vi "Clear Filters.vi"(8 "error in (no error)":errorcluster, 11 "Local Error Manager in":refnum<class "Local Error Manager.lvclass">) -> (0 "error out":errorcluster, 2 "Filters to clear":set{i32}(c389), 3 "Local Error Manager out":refnum<class "Local Error Manager.lvclass">)   [LabVIEW 2026, in "TALOS.lvlib" / "Error Manager.lvlib" / "Local Error Manager.lvclass"]
uses:
  Local Error Manager.lvclass
  Ancestor/Ancestor/Ancestor.lvclass/Ancestor.ctl
  Support VIs/Generate Error.vi
  FGV/Error Memory/Get Error Description.vi
  Support VIs/Get PC name.vi
  Ancestor/Ancestor/Read ID.vi
  Support VIs/Get Class Name.vi
  <vilib>/Utility/error.llb/Clear Errors.vi
  FGV/Error Memory/Error Memory Core.vi
  <vilib>/AdvancedString/Delimited String to 1D String Array.vi
  <vilib>/AdvancedString/Delimited String to 1D String Array (string).vi
  Support VIs/Circus Root Path.vi
  FGV/Error Memory/Error Crt Lvl checker.vi
  FGV/Error Memory/Error Memory Core.vi/40c8088d-b597-4017-91af-faa98e00292e.vi
  FGV/Error Memory/Error Memory Core.vi/d4a3ab98-063c-4e44-b43d-fbdcfe6c2be2.vi
  Support VIs/Global Memory.vi
  <vilib>/Utility/LVClass/Get LV Class Name.vi
  Support VIs/Is in Packed Library.vi
  Support VIs/TALOS Root path.vi
  Support VIs/Read CSV worksheet.vi
  Support VIs/Global Constants.vi
  <vilib>/Utility/error.llb/General Error Handler.vi
  Support VIs/Error Log.vi
  Error Manager.lvclass
  Ancestor/Ancestor/Ancestor.lvclass
  <vilib>/Comparison/Equal/Equal Functor/Equal Functor.lvclass
  TALOS.lvlib
  Classes/Error Filter/Error Filter.lvclass
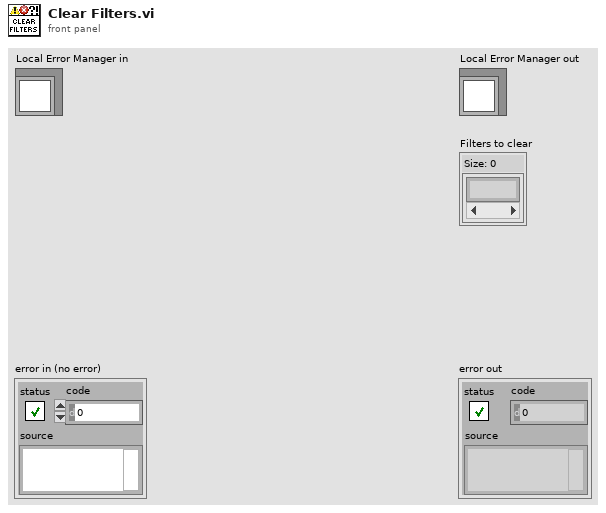
[diagram p1: front panel]
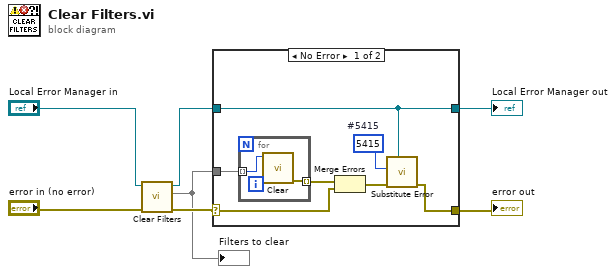
[diagram p0: block diagram]
diagram:
  n1 = call-parent "Clear Filters.vi"("error in (no error)"="error in (no error)", "Error Manager in"="Local Error Manager in") -> ("error out"=w5:errorcluster, "Filters to clear"=w4:set{i32}, "Error Manager out"=w3:refnum<class "Local Error Manager.lvclass">)  [unwired: 7 in]
  "Filters to clear" <- w4
  n2 = case shown="No Error" w5 {
    selector: w5 -> [w14 w18]
    tunnel: [w11 w18] -> w1
    tunnel: [w10 w17] -> w2
    tunnel: w3 -> [w10 w17]
    tunnel: w4 -> [w8 _]
    frame No Error {
      w13 = 5415  # #5415
      n3 = for {
        tunnel: [w16] -> w9 mode=indexing
        tunnel: w8 -> [w15] mode=indexing
        n4 = call "Clear.vi"("Error Code"=w15) -> ("error out"=w16:errorcluster)  [unwired: 10 in]
      }
      n5 = Merge Errors(w9, w14) -> (w12:errorcluster)
      n6 = call "Substitute Error.vi"("LabVIEW Object"=w10, "error in (no error)"=w12, "Error Code"=w13) -> ("error out"=w11:errorcluster)  [unwired: 8 in]
    }
    frame Error {
    }
  }
  "error out" <- w1
  "Local Error Manager out" <- w2
